vi "Current.vi"(10 "array":dbl[](array[numeric]), 11 "Flow Rate (uL/min)":dbl min=0.0 step=0.1) -> (3 "Current":dbl)   [LabVIEW 2020]
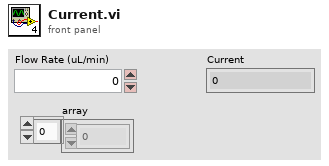
[diagram p1: front panel]
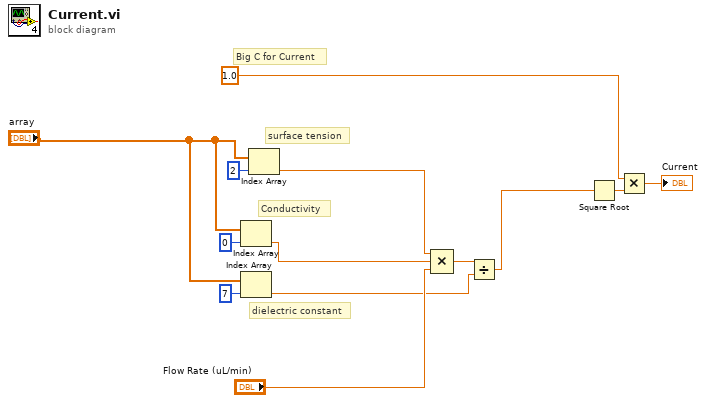
[diagram p0: block diagram]
diagram:
  # "Big C for Current"
  # "dielectric constant"
  # "Conductivity"
  # "surface tension"
  n1 = Index Array(array="array", index=0) -> (element=w9:dbl)
  n2 = Index Array(array="array", index=7) -> (element=w6:dbl)
  n3 = Index Array(array="array", index=2) -> (element=w10:dbl)
  n4 = Compound Arithmetic op=MULTIPLY(w10, w9, "Flow Rate (uL/min)") -> (w7:dbl)
  n5 = Divide(x=w7, y=w6) -> (x/y=w5:dbl)
  n6 = Square Root(x=w5) -> (sqrt(x)=w4:dbl)
  n7 = Multiply(x=1.0, y=w4) -> (x*y=→"Current":dbl)
